vi "Queues Reference.vi"(7 "Data Functions":T2, 8 "error in (no error)":errorcluster) -> (0 "error out":errorcluster, 3 "Queues Reference":T1)   [LabVIEW 2016, in "System.lvlib"]
uses:
  System.lvlib
  Controls/Control_Data Functions.ctl
  Controls/Control_Variant Data Reference.ctl
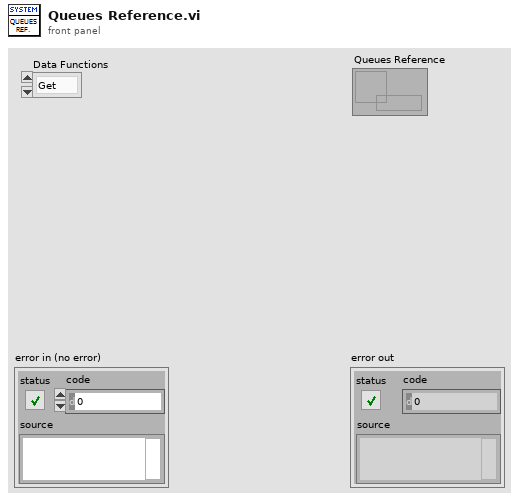
[diagram p1: front panel]
types:
  T1 = typedef "System.lvlib/Control_Variant Data Reference.ctl" = refnum<data-value>
  T2 = typedef "System.lvlib/Control_Data Functions.ctl" = enum16{"Get", "Set", "Release"}
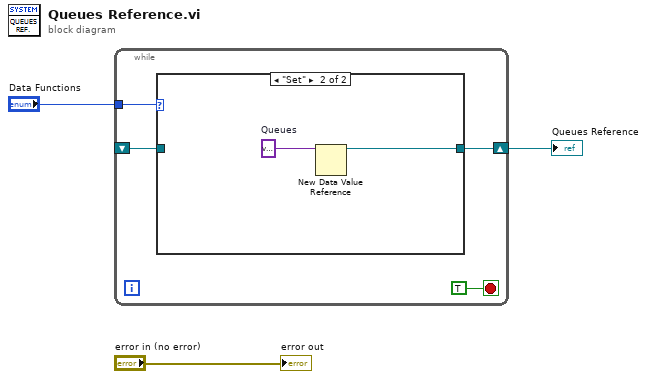
[diagram p0: block diagram]
diagram:
  n1 = while {
    tunnel: "Data Functions" -> [w6]
    shift-right: [w5] -> w2
    shift-left: _ -> [w4]
    stop <- TRUE stop-if-true
    n2 = case shown="\"Set\"" w6 {
      tunnel: [w8 w10] -> w5
      tunnel: w4 -> [w8 _]
      frame "Get", Default {
      }
      frame "Set" {
        w9 = variant  # Queues
        n3 = New Data Value Reference(data value=w9) -> (data value reference=w10:refnum<data-value>)  [unwired: 1 in, 1 out]
      }
    }
  }
  "Queues Reference" <- w2
  "error out" <- "error in (no error)"
